vi "GUI.vi"(8 "error in (no error)":errorcluster) -> (0 "error out":errorcluster)   [LabVIEW 2017]
uses:
  Type Definitions/Queue FG Options.ctl
  Type Definitions/GUI Data.ctl
  Type Definitions/Controller States.ctl
  Type Definitions/Controller Message.ctl
  Type Definitions/Controller Data.ctl
  Type Definitions/DB Data.ctl
  Type Definitions/DB Info.ctl
  Type Definitions/Display Data.ctl
  Type Definitions/DB Record.ctl
  Type Definitions/Display Console States.ctl
  Type Definitions/Sensor UI Data.ctl
  Current State.vi
panel:
  in  "stop":bool
  in  "Transactions":T1
  in  "Pinpad":T2
  in  "Card Reader":bool
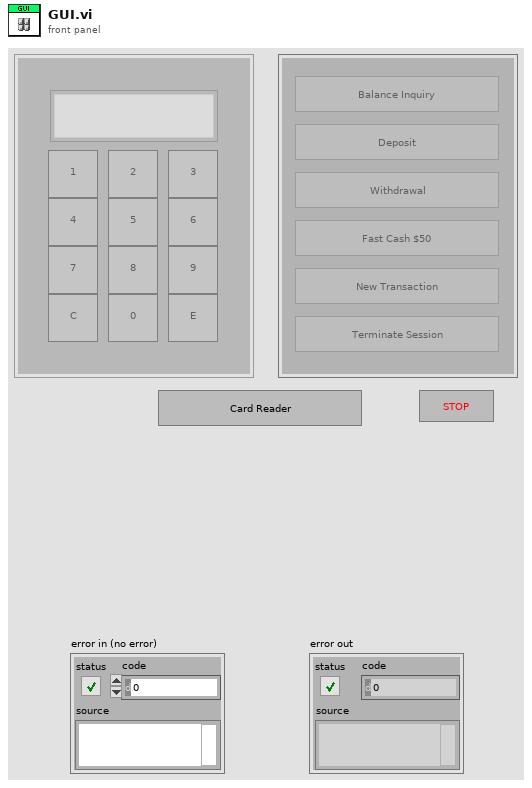
[diagram p1: front panel]
types:
  T1 = cluster{"Balance Inquiry":bool, "Deposit":bool, "Withdrawal":bool, "Fast Cash $50":bool, "New Transaction":bool, "Terminate Session":bool}
  T2 = cluster{"Screen":string, "num1":bool, "num2":bool, "num3":bool, "num6":bool, "num5":bool, "num4":bool, "num7":bool, "num8":bool, "num9":bool, "C":bool, "num0":bool, "E":bool}
  T3 = typedef "Queue FG Options.ctl" = enum16{"Set", "Get", "Read", "Write", "Destroy"}
  T4 = typedef "GUI Data.ctl" = cluster{"Card Reader":enum8{"Enabled", "Disabled", "Disabled and Grayed Out"}, "Keypad":enum8{"Enabled", "Disabled", "Disabled and Grayed Out"}, "Balance Inquiry":enum8{"Enabled", "Disabled", "Disabled and Grayed Out"}, "Deposit":enum8{"Enabled", "Disabled", "Disabled and Grayed Out"}, "Withdrawal":enum8{"Enabled", "Disabled", "Disabled and Grayed Out"}, "Fast Cash":enum8{"Enabled", "Disabled", "Disabled and Grayed Out"}, "New Transaction":enum8{"Enabled", "Disabled", "Disabled and Grayed Out"}, "Terminate Session":enum8{"Enabled", "Disabled", "Disabled and Grayed Out"}, "Pinpad Value":string, "Timeout":i32, "Controller States":T5}
  T5 = typedef "Controller States.ctl" = enum16{"Timeout", "Initial", "Login", "Idle", "Balance Inquiry", "Deposit", "Withdrawal", "Fast Cash", "Terminate", "Wait on Exit", "Shutdown", "Error Handler"}
  T6 = typedef "DB Info.ctl" = enum16{"Empty", "Verify", "Login Accepted", "Invalid Login", "Deposit Complete", "Withdrawal Complete", "Withdrawal Failed", "Terminate"}
  T7 = typedef "Controller Data.ctl" = cluster{"Time":dbl, "DB Data in":T8, "Display Data":T9, "GUI Data ":T4, "Sensor UI":T12, "Controller States":T5}
  T8 = typedef "DB Data.ctl" = cluster{"Account":i32, "First Name":string, "Last Name":string, "Balance":fxp<+/-,64,35>, "DB Info":T6}
  T9 = typedef "Display Data.ctl" = cluster{"Message Text":string, "DB Record":T10, "Card Read":bool, "Display Console States":T11}
  T10 = typedef "DB Record.ctl" = cluster{"Account":i32, "First Name":string, "Last Name":string, "Balance":fxp<+/-,64,35>}
  T11 = typedef "Display Console States.ctl" = enum16{"Timeout", "Initial", "Login", "Invalid Login", "Idle", "Balance Inquiry", "Deposit", "Withdrawal", "Fast Cash", "Withdrawal Failed", "Withdrawal Complete", "Terminate", "Shutdown"}
  T12 = typedef "Sensor UI Data.ctl" = cluster{"Funds dispensed":enum16{"Enabled", "Disabled", "Disabled and Grayed Out"}, "Deposit received":enum16{"Enabled", "Disabled", "Disabled and Grayed Out"}, "Timeout":dbl}
  T13 = typedef "Controller Message.ctl" = cluster{"Message Info":T5, "Message Data":variant}
  T14 = enum8{"Enabled", "Disabled", "Disabled and Grayed Out"}
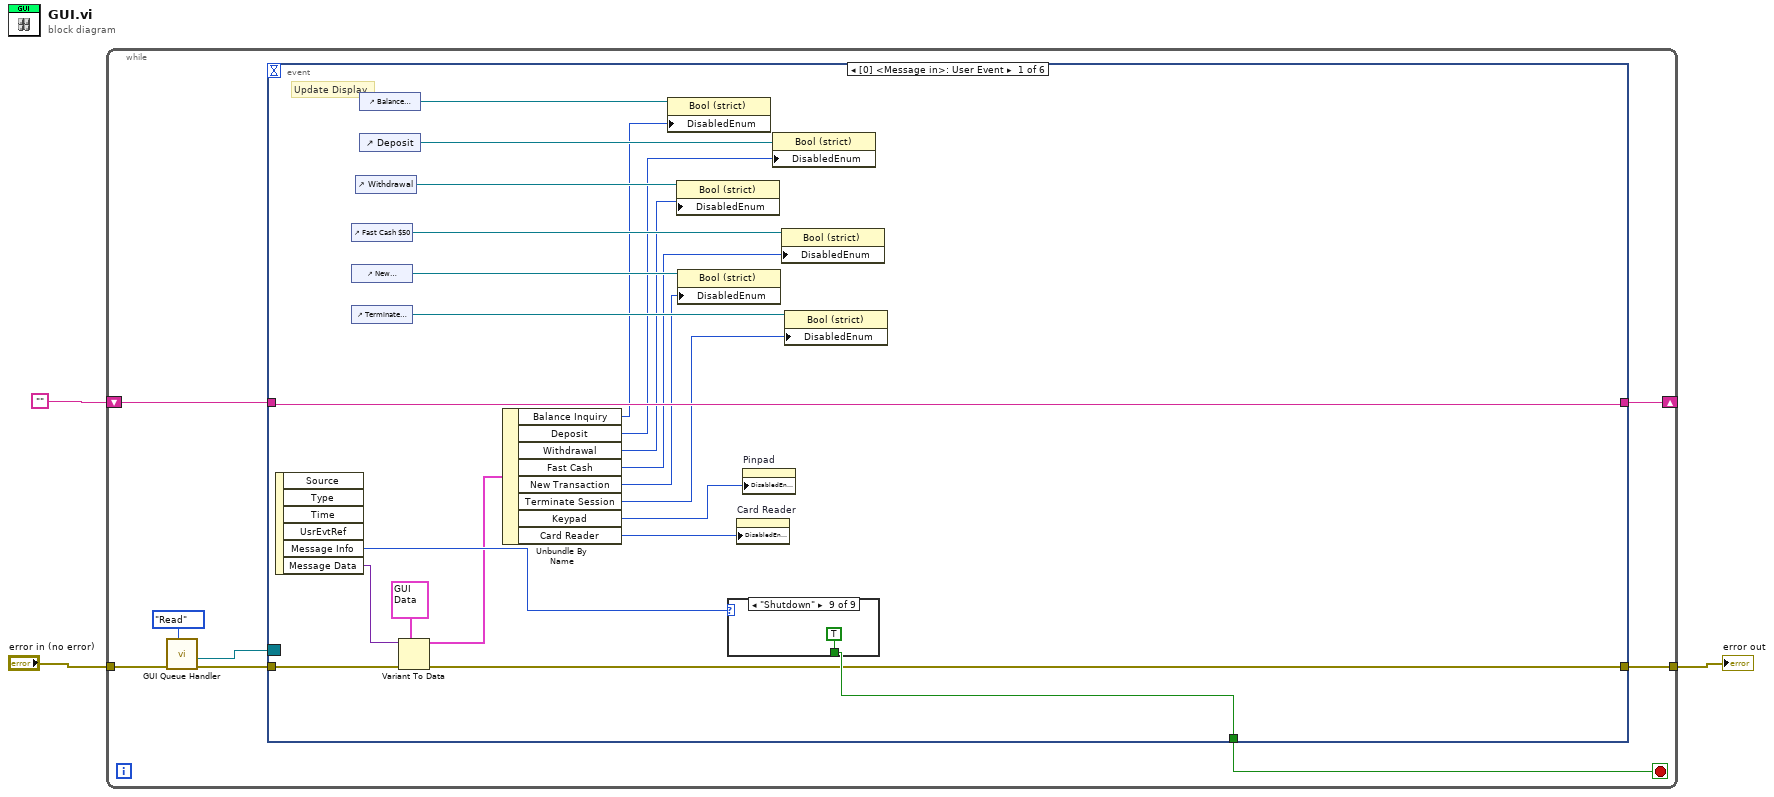
[diagram p0: block diagram]
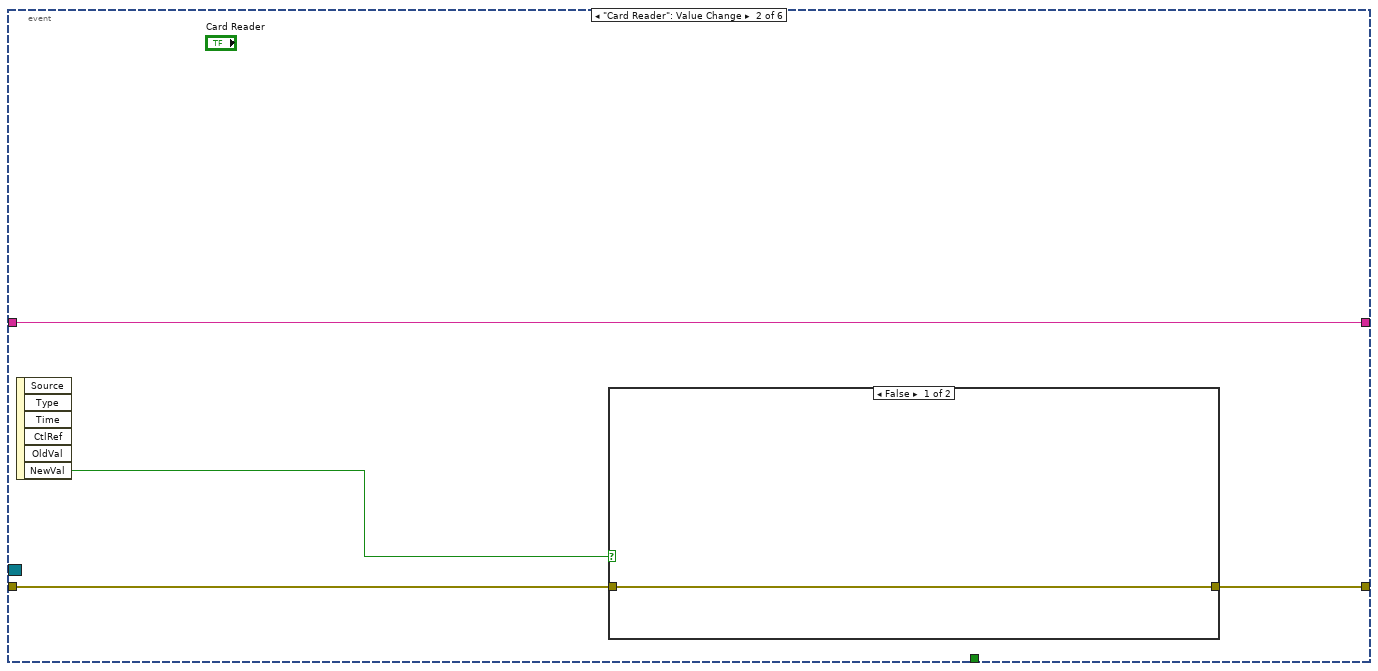
[diagram p10: hidden frame]
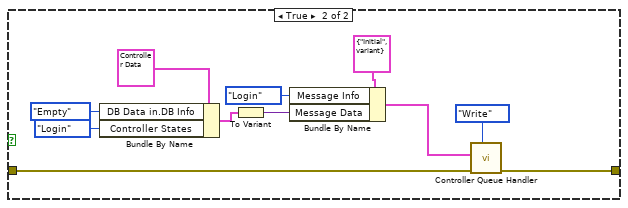
[diagram p11: hidden frame]
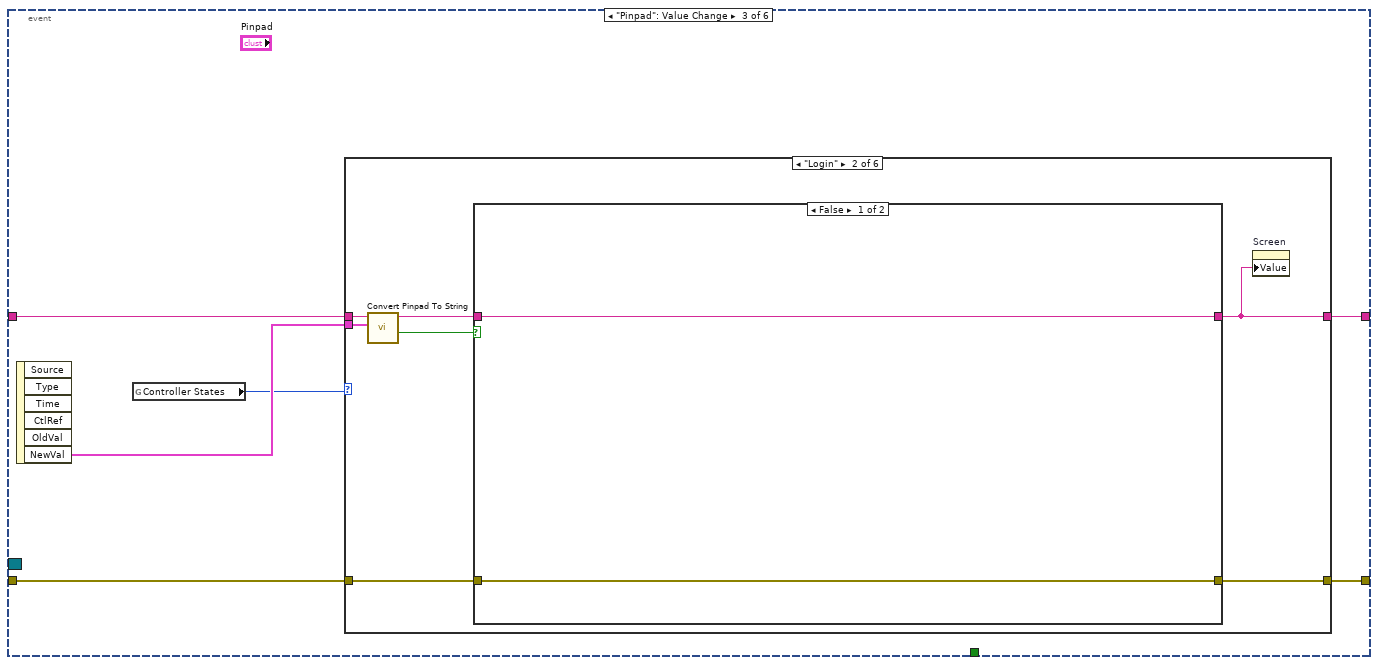
[diagram p12: hidden frame]
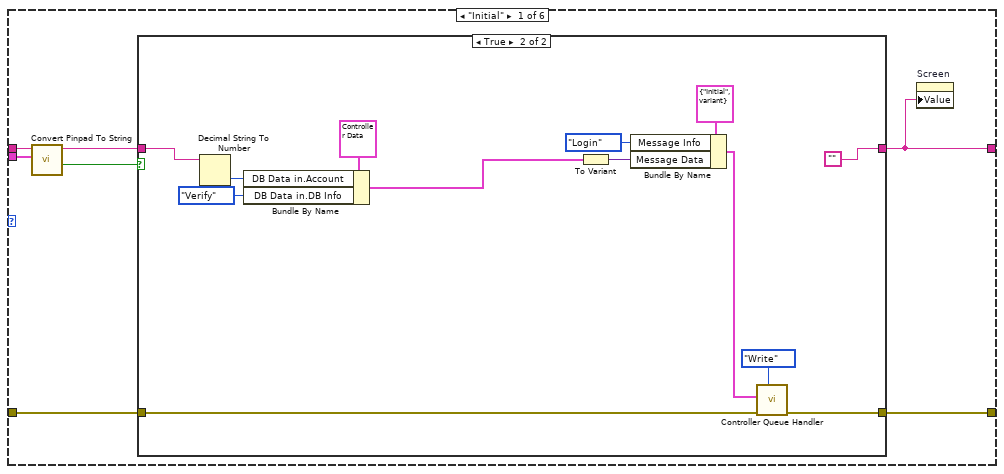
[diagram p13: hidden frame]
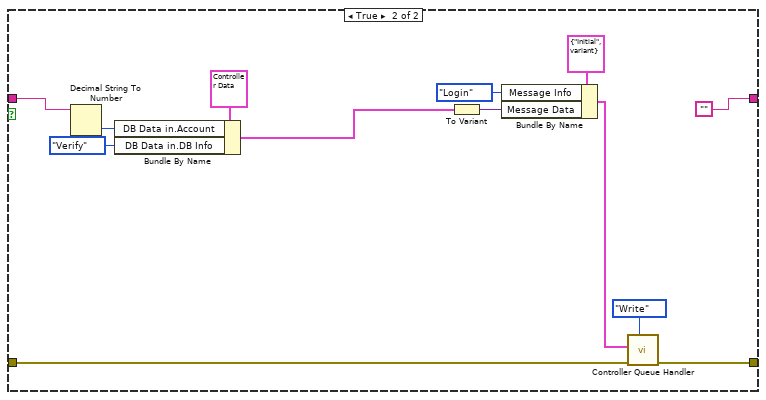
[diagram p15: hidden frame]
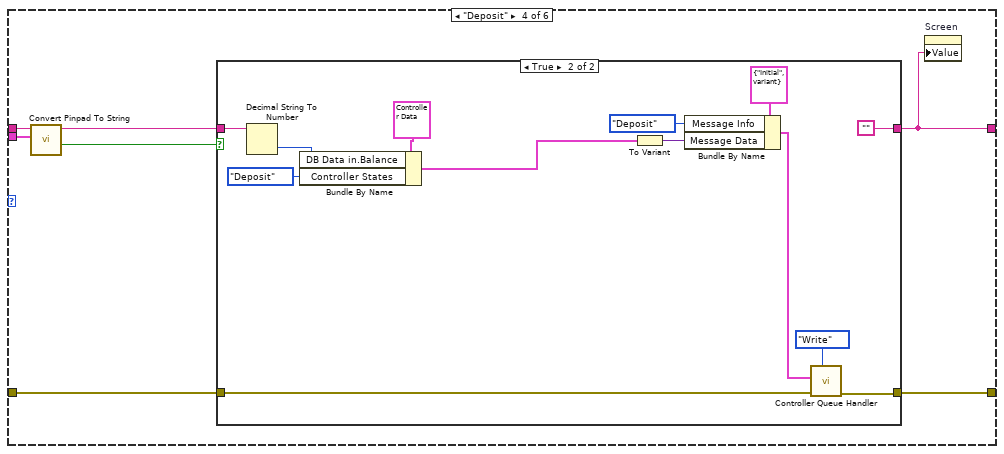
[diagram p17: hidden frame]
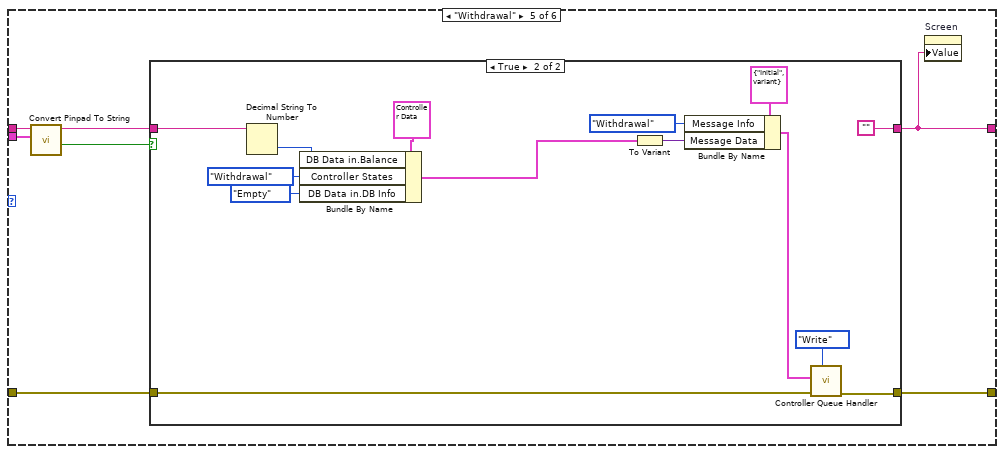
[diagram p19: hidden frame]
diagram:
  n1 = while {
    tunnel: "error in (no error)" -> [w6]
    tunnel: [w9] -> w2
    shift-right: [w7] -> _
    shift-left: "" -> [w8]
    stop <- w4 stop-if-true
    n2 = call "GUI Queue Handler.vi"("Action"=Queue_FG_Options."Read", "error in (no error)"=w6) -> ("error out"=w10:errorcluster, "Event Registration Refnum"=w5:refnum<event-registration>)  [unwired: 6 in, 2 out]
    n3 = event shown="[0] <Message in>: User Event" {
      selector: w5 -> [_ _ _ _ _ _]
      dyn-events: _ -> [_ _ _ _ _ _]
      timeout: _ -> [_ _ _ _ _ _]
      tunnel: w10 -> [w32 w37 w56 w157 w171 w240]
      tunnel: [w29 w36 w55 w154 w170 w240] -> w9
      tunnel: w8 -> [w33 w38 w54 w156 w169 w239]
      tunnel: [w33 w38 w53 w156 w168 w239] -> w7
      tunnel: [w30 _ _ TRUE _ _] -> w4
      event User Event {
        # "Update Display"
        n4 = event-data() -> ("Message Info"=w31:T5, "Message Data"=w28:variant)  [unwired: 1 in, 4 out]
        n5 = control-ref of="Fast Cash $50"() -> (w22:refnum<vi>)
        n6 = control-ref of="New Transaction"() -> (w21:refnum<vi>)
        n7 = control-ref of="Terminate Session"() -> (w20:refnum<vi>)
        n8 = control-ref of="Withdrawal"() -> (w19:refnum<vi>)
        n9 = control-ref of="Balance Inquiry"() -> (w24:refnum<vi>)
        n10 = control-ref of="Deposit"() -> (w23:refnum<vi>)
        n11 = Variant To Data(error in=w32, type=T4 {"Card Reader"=enum."Enabled", "Keypad"=enum."Enabled", "Balance Inquiry"=enum."Enabled", "Deposit"=enum."Enabled", "Withdrawal"=enum."Enabled", "Fast Cash"=enum."Enabled", "New Transaction"=enum."Enabled", "Terminate Session"=enum."Enabled", "Pinpad Value"="", "Timeout"=0, "Controller States"=enum."Initial"} ("GUI Data"), Variant=w28) -> (data=w26:T4, error out=w29:errorcluster)
        n12 = Unbundle By Name(w26) -> ("Balance Inquiry"=w17:T14, "Deposit"=w16:T14, "Withdrawal"=w14:T14, "Fast Cash"=w15:T14, "New Transaction"=w13:T14, "Terminate Session"=w12:T14, "Keypad"=w18:T14, "Card Reader"=w25:T14)
        n13 = property class="Bool (strict)"(reference=w24, "DisabledEnum"=w17) -> ()  [unwired: 1 in, 2 out]
        n14 = property class="Bool (strict)"(reference=w19, "DisabledEnum"=w14) -> ()  [unwired: 1 in, 2 out]
        n15 = property class="Bool (strict)"(reference=w21, "DisabledEnum"=w13) -> ()  [unwired: 1 in, 2 out]
        n16 = case shown="\"Shutdown\"" w31 {
          tunnel: [_ _ _ _ _ _ _ _ TRUE] -> w30
          frame "Initial", Default {
          }
          frame "Login" {
          }
          frame "Idle" {
          }
          frame "Balance Inquiry" {
          }
          frame "Deposit" {
          }
          frame "Withdrawal" {
          }
          frame "Fast Cash" {
          }
          frame "Terminate" {
          }
          frame "Shutdown" {
          }
        }
        n17 = property on="Card Reader" class="Bool"("DisabledEnum"=w25) -> ()  [unwired: 2 in, 2 out]
        n18 = property on="Pinpad" class="Clust (strict)"("DisabledEnum"=w18) -> ()  [unwired: 2 in, 2 out]
        n19 = property class="Bool (strict)"(reference=w23, "DisabledEnum"=w16) -> ()  [unwired: 1 in, 2 out]
        n20 = property class="Bool (strict)"(reference=w22, "DisabledEnum"=w15) -> ()  [unwired: 1 in, 2 out]
        n21 = property class="Bool (strict)"(reference=w20, "DisabledEnum"=w12) -> ()  [unwired: 1 in, 2 out]
      }
      event "Card Reader": Value Change {
        n22 = event-data() -> ("NewVal"=w35:bool)  [unwired: 1 in, 5 out]
        n23 = case shown="False" w35 {
          tunnel: w37 -> [w39 w50]
          tunnel: [w39 w49] -> w36
          frame False {
          }
          frame True {
            n24 = Bundle By Name(cluster=T7 {"Time"=0.0, "DB Data in"={"Account"=0, "First Name"="", "Last Name"="", "Balance"=0.0, "DB Info"=enum."Login Accepted"}, "Display Data"={"Message Text"="", "DB Record"={"Account"=0, "First Name"="", "Last Name"="", "Balance"=0.0}, "Card Read"=FALSE, "Display Console States"=enum."Timeout"}, "GUI Data "={"Card Reader"=enum."Enabled", "Keypad"=enum."Enabled", "Balance Inquiry"=enum."Enabled", "Deposit"=enum."Enabled", "Withdrawal"=enum."Enabled", "Fast Cash"=enum."Enabled", "New Transaction"=enum."Enabled", "Terminate Session"=enum."Enabled", "Pinpad Value"="", "Timeout"=0, "Controller States"=enum."Initial"}, "Sensor UI"={"Funds dispensed"=enum."Enabled", "Deposit received"=enum."Enabled", "Timeout"=0.0}, "Controller States"=enum."Timeout"} ("Controller Data"), "DB Data in.DB Info"=DB_Info."Empty", "Controller States"=Controller_States."Login") -> (w43:T7)
            n25 = To Variant(anything=w43) -> (Variant=w42:variant)
            n26 = Bundle By Name(cluster=T13 {"Message Info"=enum."Initial", "Message Data"=variant} ("Message"), "Message Info"=Controller_States."Login", "Message Data"=w42) -> (w45:T13)
            n27 = call "Controller Queue Handler.vi"("Action"=Queue_FG_Options."Write", "error in (no error)"=w50, "Message in"=w45) -> ("error out"=w49:errorcluster)  [unwired: 6 in, 2 out]
          }
        }
      }
      event "Pinpad": Value Change {
        n28 = event-data() -> ("NewVal"=w52:T2)  [unwired: 1 in, 5 out]
        n29 = global read "Current State.vi" "Controller States"() -> (w51:T5)
        n30 = case shown="\"Login\"" w51 {
          tunnel: w56 -> [w63 w85 w102 w106 w128 w149]
          tunnel: [w62 w84 w102 w105 w127 w149] -> w55
          tunnel: w54 -> [w61 w83 w101 w108 w130 w148]
          tunnel: [w59 w81 w101 w103 w125 w148] -> w53
          tunnel: w52 -> [w57 w79 _ w109 w131 _]
          frame "Initial" {
            n31 = call "Convert Pinpad To String.vi"("Pinpad"=w57, "Screen in"=w61) -> ("E"=w58:bool, "Screen out"=w60:string)  [unwired: 8 in]
            n32 = case shown="True" w58 {
              tunnel: w63 -> [w65 w76]
              tunnel: [w65 w73] -> w62
              tunnel: w60 -> [w64 w69]
              tunnel: [w64 ""] -> w59
              frame False {
              }
              frame True {
                n33 = Decimal String To Number(string=w69) -> (number=w68:i32)  [unwired: 2 in, 1 out]
                n34 = Bundle By Name(cluster=T7 {"Time"=0.0, "DB Data in"={"Account"=0, "First Name"="", "Last Name"="", "Balance"=0.0, "DB Info"=enum."Login Accepted"}, "Display Data"={"Message Text"="", "DB Record"={"Account"=0, "First Name"="", "Last Name"="", "Balance"=0.0}, "Card Read"=FALSE, "Display Console States"=enum."Timeout"}, "GUI Data "={"Card Reader"=enum."Enabled", "Keypad"=enum."Enabled", "Balance Inquiry"=enum."Enabled", "Deposit"=enum."Enabled", "Withdrawal"=enum."Enabled", "Fast Cash"=enum."Enabled", "New Transaction"=enum."Enabled", "Terminate Session"=enum."Enabled", "Pinpad Value"="", "Timeout"=0, "Controller States"=enum."Initial"}, "Sensor UI"={"Funds dispensed"=enum."Enabled", "Deposit received"=enum."Enabled", "Timeout"=0.0}, "Controller States"=enum."Timeout"} ("Controller Data"), "DB Data in.Account"=w68, "DB Data in.DB Info"=DB_Info."Verify") -> (w67:T7)
                n35 = To Variant(anything=w67) -> (Variant=w77:variant)
                n36 = Bundle By Name(cluster=T13 {"Message Info"=enum."Initial", "Message Data"=variant} ("Message"), "Message Info"=Controller_States."Login", "Message Data"=w77) -> (w71:T13)
                n37 = call "Controller Queue Handler.vi"("Action"=Queue_FG_Options."Write", "error in (no error)"=w76, "Message in"=w71) -> ("error out"=w73:errorcluster)  [unwired: 6 in, 2 out]
              }
            }
            n38 = property on="Screen" class="Str"("Value"=w59) -> ()  [unwired: 2 in, 2 out]
          }
          frame "Login" {
            n39 = call "Convert Pinpad To String.vi"("Pinpad"=w79, "Screen in"=w83) -> ("E"=w80:bool, "Screen out"=w82:string)  [unwired: 8 in]
            n40 = case shown="False" w80 {
              tunnel: w85 -> [w87 w98]
              tunnel: [w87 w95] -> w84
              tunnel: w82 -> [w86 w91]
              tunnel: [w86 ""] -> w81
              frame False {
              }
              frame True {
                n41 = Decimal String To Number(string=w91) -> (number=w90:i32)  [unwired: 2 in, 1 out]
                n42 = Bundle By Name(cluster=T7 {"Time"=0.0, "DB Data in"={"Account"=0, "First Name"="", "Last Name"="", "Balance"=0.0, "DB Info"=enum."Login Accepted"}, "Display Data"={"Message Text"="", "DB Record"={"Account"=0, "First Name"="", "Last Name"="", "Balance"=0.0}, "Card Read"=FALSE, "Display Console States"=enum."Timeout"}, "GUI Data "={"Card Reader"=enum."Enabled", "Keypad"=enum."Enabled", "Balance Inquiry"=enum."Enabled", "Deposit"=enum."Enabled", "Withdrawal"=enum."Enabled", "Fast Cash"=enum."Enabled", "New Transaction"=enum."Enabled", "Terminate Session"=enum."Enabled", "Pinpad Value"="", "Timeout"=0, "Controller States"=enum."Initial"}, "Sensor UI"={"Funds dispensed"=enum."Enabled", "Deposit received"=enum."Enabled", "Timeout"=0.0}, "Controller States"=enum."Timeout"} ("Controller Data"), "DB Data in.Account"=w90, "DB Data in.DB Info"=DB_Info."Verify") -> (w89:T7)
                n43 = To Variant(anything=w89) -> (Variant=w99:variant)
                n44 = Bundle By Name(cluster=T13 {"Message Info"=enum."Initial", "Message Data"=variant} ("Message"), "Message Info"=Controller_States."Login", "Message Data"=w99) -> (w93:T13)
                n45 = call "Controller Queue Handler.vi"("Action"=Queue_FG_Options."Write", "error in (no error)"=w98, "Message in"=w93) -> ("error out"=w95:errorcluster)  [unwired: 6 in, 2 out]
              }
            }
            n46 = property on="Screen" class="Str"("Value"=w81) -> ()  [unwired: 2 in, 2 out]
          }
          frame "Idle", Default {
          }
          frame "Deposit" {
            n47 = call "Convert Pinpad To String.vi"("Pinpad"=w109, "Screen in"=w108) -> ("E"=w107:bool, "Screen out"=w104:string)  [unwired: 8 in]
            n48 = case shown="True" w107 {
              tunnel: w106 -> [w110 w115]
              tunnel: [w110 w114] -> w105
              tunnel: w104 -> [w111 w116]
              tunnel: [w111 ""] -> w103
              frame False {
              }
              frame True {
                n49 = Decimal String To Number(string=w116) -> (number=w118:i32)  [unwired: 2 in, 1 out]
                n50 = Bundle By Name(cluster=T7 {"Time"=0.0, "DB Data in"={"Account"=0, "First Name"="", "Last Name"="", "Balance"=0.0, "DB Info"=enum."Login Accepted"}, "Display Data"={"Message Text"="", "DB Record"={"Account"=0, "First Name"="", "Last Name"="", "Balance"=0.0}, "Card Read"=FALSE, "Display Console States"=enum."Timeout"}, "GUI Data "={"Card Reader"=enum."Enabled", "Keypad"=enum."Enabled", "Balance Inquiry"=enum."Enabled", "Deposit"=enum."Enabled", "Withdrawal"=enum."Enabled", "Fast Cash"=enum."Enabled", "New Transaction"=enum."Enabled", "Terminate Session"=enum."Enabled", "Pinpad Value"="", "Timeout"=0, "Controller States"=enum."Initial"}, "Sensor UI"={"Funds dispensed"=enum."Enabled", "Deposit received"=enum."Enabled", "Timeout"=0.0}, "Controller States"=enum."Timeout"} ("Controller Data"), "DB Data in.Balance"=w118, "Controller States"=Controller_States."Deposit") -> (w117:T7)
                n51 = To Variant(anything=w117) -> (Variant=w123:variant)
                n52 = Bundle By Name(cluster=T13 {"Message Info"=enum."Initial", "Message Data"=variant} ("Message"), "Message Info"=Controller_States."Deposit", "Message Data"=w123) -> (w120:T13)
                n53 = call "Controller Queue Handler.vi"("Action"=Queue_FG_Options."Write", "error in (no error)"=w115, "Message in"=w120) -> ("error out"=w114:errorcluster)  [unwired: 6 in, 2 out]
              }
            }
            n54 = property on="Screen" class="Str"("Value"=w103) -> ()  [unwired: 2 in, 2 out]
          }
          frame "Withdrawal" {
            n55 = call "Convert Pinpad To String.vi"("Pinpad"=w131, "Screen in"=w130) -> ("E"=w129:bool, "Screen out"=w126:string)  [unwired: 8 in]
            n56 = case shown="True" w129 {
              tunnel: w128 -> [w132 w138]
              tunnel: [w132 w137] -> w127
              tunnel: w126 -> [w133 w139]
              tunnel: [w133 ""] -> w125
              frame False {
              }
              frame True {
                n57 = Decimal String To Number(string=w139) -> (number=w141:i32)  [unwired: 2 in, 1 out]
                n58 = Bundle By Name(cluster=T7 {"Time"=0.0, "DB Data in"={"Account"=0, "First Name"="", "Last Name"="", "Balance"=0.0, "DB Info"=enum."Login Accepted"}, "Display Data"={"Message Text"="", "DB Record"={"Account"=0, "First Name"="", "Last Name"="", "Balance"=0.0}, "Card Read"=FALSE, "Display Console States"=enum."Timeout"}, "GUI Data "={"Card Reader"=enum."Enabled", "Keypad"=enum."Enabled", "Balance Inquiry"=enum."Enabled", "Deposit"=enum."Enabled", "Withdrawal"=enum."Enabled", "Fast Cash"=enum."Enabled", "New Transaction"=enum."Enabled", "Terminate Session"=enum."Enabled", "Pinpad Value"="", "Timeout"=0, "Controller States"=enum."Initial"}, "Sensor UI"={"Funds dispensed"=enum."Enabled", "Deposit received"=enum."Enabled", "Timeout"=0.0}, "Controller States"=enum."Timeout"} ("Controller Data"), "DB Data in.Balance"=w141, "Controller States"=Controller_States."Withdrawal", "DB Data in.DB Info"=DB_Info."Empty") -> (w140:T7)
                n59 = To Variant(anything=w140) -> (Variant=w146:variant)
                n60 = Bundle By Name(cluster=T13 {"Message Info"=enum."Initial", "Message Data"=variant} ("Message"), "Message Info"=Controller_States."Withdrawal", "Message Data"=w146) -> (w143:T13)
                n61 = call "Controller Queue Handler.vi"("Action"=Queue_FG_Options."Write", "error in (no error)"=w138, "Message in"=w143) -> ("error out"=w137:errorcluster)  [unwired: 6 in, 2 out]
              }
            }
            n62 = property on="Screen" class="Str"("Value"=w125) -> ()  [unwired: 2 in, 2 out]
          }
          frame "Balance Inquiry" {
          }
        }
      }
      event "stop": Value Change {
        n63 = event-data() -> ()  [unwired: 1 in, 6 out]
        n64 = Bundle By Name(cluster=T13 {"Message Info"=enum."Initial", "Message Data"=variant} ("Message"), "Message Info"=Controller_States."Wait on Exit" ("Controller States")) -> (w151:T13)
        n65 = call "Controller Queue Handler.vi"("Action"=Queue_FG_Options."Write", "error in (no error)"=w157, "Message in"=w151) -> ("error out"=w154:errorcluster)  [unwired: 6 in, 2 out]
      }
      event "Transactions": Value Change {
        n66 = event-data() -> ("OldVal"=w158:T1, "NewVal"=w167:T1)  [unwired: 1 in, 4 out]
        n67 = Cluster To Array(cluster=w158) -> (array=w164:bool[])
        n68 = Cluster To Array(cluster=w167) -> (array=w166:bool[])
        n69 = Search 1D Array(1D array=w164, element=TRUE) -> (index of element=w161:i32)  [unwired: 1 in]
        n70 = Search 1D Array(1D array=w166, element=TRUE) -> (index of element=w159:i32)  [unwired: 1 in]
        n71 = Equal?(x=w159, y=-1) -> (x = y?=w162:bool)
        n72 = Select(t=w161, s=w162, f=w159) -> (s? t:f=w160:i32)
        n73 = case shown="1" w160 {
          tunnel: w171 -> [w183 w194 w205 w216 w227 w238]
          tunnel: [w181 w192 w203 w214 w225 w236] -> w170
          tunnel: w169 -> [w182 w193 w204 w215 w226 w237]
          tunnel: [w182 w193 w204 w215 w226 w237] -> w168
          frame 0, Default {
            n74 = Bundle By Name(cluster=T7 {"Time"=0.0, "DB Data in"={"Account"=0, "First Name"="", "Last Name"="", "Balance"=0.0, "DB Info"=enum."Login Accepted"}, "Display Data"={"Message Text"="", "DB Record"={"Account"=0, "First Name"="", "Last Name"="", "Balance"=0.0}, "Card Read"=FALSE, "Display Console States"=enum."Timeout"}, "GUI Data "={"Card Reader"=enum."Enabled", "Keypad"=enum."Enabled", "Balance Inquiry"=enum."Enabled", "Deposit"=enum."Enabled", "Withdrawal"=enum."Enabled", "Fast Cash"=enum."Enabled", "New Transaction"=enum."Enabled", "Terminate Session"=enum."Enabled", "Pinpad Value"="", "Timeout"=0, "Controller States"=enum."Initial"}, "Sensor UI"={"Funds dispensed"=enum."Enabled", "Deposit received"=enum."Enabled", "Timeout"=0.0}, "Controller States"=enum."Timeout"} ("Controller Data"), "Controller States"=Controller_States."Balance Inquiry") -> (w174:T7)
            n75 = To Variant(anything=w174) -> (Variant=w173:variant)
            n76 = Bundle By Name(cluster=T13 {"Message Info"=enum."Initial", "Message Data"=variant} ("Message"), "Message Info"=Controller_States."Balance Inquiry", "Message Data"=w173) -> (w178:T13)
            n77 = call "Controller Queue Handler.vi"("Action"=Queue_FG_Options."Write", "error in (no error)"=w183, "Message in"=w178) -> ("error out"=w181:errorcluster)  [unwired: 6 in, 2 out]
          }
          frame 1 {
            n78 = Bundle By Name(cluster=T7 {"Time"=0.0, "DB Data in"={"Account"=0, "First Name"="", "Last Name"="", "Balance"=0.0, "DB Info"=enum."Login Accepted"}, "Display Data"={"Message Text"="", "DB Record"={"Account"=0, "First Name"="", "Last Name"="", "Balance"=0.0}, "Card Read"=FALSE, "Display Console States"=enum."Timeout"}, "GUI Data "={"Card Reader"=enum."Enabled", "Keypad"=enum."Enabled", "Balance Inquiry"=enum."Enabled", "Deposit"=enum."Enabled", "Withdrawal"=enum."Enabled", "Fast Cash"=enum."Enabled", "New Transaction"=enum."Enabled", "Terminate Session"=enum."Enabled", "Pinpad Value"="", "Timeout"=0, "Controller States"=enum."Initial"}, "Sensor UI"={"Funds dispensed"=enum."Enabled", "Deposit received"=enum."Enabled", "Timeout"=0.0}, "Controller States"=enum."Timeout"} ("Controller Data"), "Controller States"=Controller_States."Deposit") -> (w185:T7)
            n79 = To Variant(anything=w185) -> (Variant=w184:variant)
            n80 = Bundle By Name(cluster=T13 {"Message Info"=enum."Initial", "Message Data"=variant} ("Message"), "Message Info"=Controller_States."Deposit", "Message Data"=w184) -> (w189:T13)
            n81 = call "Controller Queue Handler.vi"("Action"=Queue_FG_Options."Write", "error in (no error)"=w194, "Message in"=w189) -> ("error out"=w192:errorcluster)  [unwired: 6 in, 2 out]
          }
          frame 2 {
            n82 = Bundle By Name(cluster=T7 {"Time"=0.0, "DB Data in"={"Account"=0, "First Name"="", "Last Name"="", "Balance"=0.0, "DB Info"=enum."Login Accepted"}, "Display Data"={"Message Text"="", "DB Record"={"Account"=0, "First Name"="", "Last Name"="", "Balance"=0.0}, "Card Read"=FALSE, "Display Console States"=enum."Timeout"}, "GUI Data "={"Card Reader"=enum."Enabled", "Keypad"=enum."Enabled", "Balance Inquiry"=enum."Enabled", "Deposit"=enum."Enabled", "Withdrawal"=enum."Enabled", "Fast Cash"=enum."Enabled", "New Transaction"=enum."Enabled", "Terminate Session"=enum."Enabled", "Pinpad Value"="", "Timeout"=0, "Controller States"=enum."Initial"}, "Sensor UI"={"Funds dispensed"=enum."Enabled", "Deposit received"=enum."Enabled", "Timeout"=0.0}, "Controller States"=enum."Timeout"} ("Controller Data"), "Controller States"=Controller_States."Withdrawal") -> (w196:T7)
            n83 = To Variant(anything=w196) -> (Variant=w195:variant)
            n84 = Bundle By Name(cluster=T13 {"Message Info"=enum."Initial", "Message Data"=variant} ("Message"), "Message Info"=Controller_States."Withdrawal", "Message Data"=w195) -> (w200:T13)
            n85 = call "Controller Queue Handler.vi"("Action"=Queue_FG_Options."Write", "error in (no error)"=w205, "Message in"=w200) -> ("error out"=w203:errorcluster)  [unwired: 6 in, 2 out]
          }
          frame 3 {
            n86 = Bundle By Name(cluster=T7 {"Time"=0.0, "DB Data in"={"Account"=0, "First Name"="", "Last Name"="", "Balance"=0.0, "DB Info"=enum."Login Accepted"}, "Display Data"={"Message Text"="", "DB Record"={"Account"=0, "First Name"="", "Last Name"="", "Balance"=0.0}, "Card Read"=FALSE, "Display Console States"=enum."Timeout"}, "GUI Data "={"Card Reader"=enum."Enabled", "Keypad"=enum."Enabled", "Balance Inquiry"=enum."Enabled", "Deposit"=enum."Enabled", "Withdrawal"=enum."Enabled", "Fast Cash"=enum."Enabled", "New Transaction"=enum."Enabled", "Terminate Session"=enum."Enabled", "Pinpad Value"="", "Timeout"=0, "Controller States"=enum."Initial"}, "Sensor UI"={"Funds dispensed"=enum."Enabled", "Deposit received"=enum."Enabled", "Timeout"=0.0}, "Controller States"=enum."Timeout"} ("Controller Data"), "Controller States"=Controller_States."Fast Cash") -> (w207:T7)
            n87 = To Variant(anything=w207) -> (Variant=w206:variant)
            n88 = Bundle By Name(cluster=T13 {"Message Info"=enum."Initial", "Message Data"=variant} ("Message"), "Message Info"=Controller_States."Fast Cash", "Message Data"=w206) -> (w211:T13)
            n89 = call "Controller Queue Handler.vi"("Action"=Queue_FG_Options."Write", "error in (no error)"=w216, "Message in"=w211) -> ("error out"=w214:errorcluster)  [unwired: 6 in, 2 out]
          }
          frame 4 {
            n90 = Bundle By Name(cluster=T7 {"Time"=0.0, "DB Data in"={"Account"=0, "First Name"="", "Last Name"="", "Balance"=0.0, "DB Info"=enum."Login Accepted"}, "Display Data"={"Message Text"="", "DB Record"={"Account"=0, "First Name"="", "Last Name"="", "Balance"=0.0}, "Card Read"=FALSE, "Display Console States"=enum."Timeout"}, "GUI Data "={"Card Reader"=enum."Enabled", "Keypad"=enum."Enabled", "Balance Inquiry"=enum."Enabled", "Deposit"=enum."Enabled", "Withdrawal"=enum."Enabled", "Fast Cash"=enum."Enabled", "New Transaction"=enum."Enabled", "Terminate Session"=enum."Enabled", "Pinpad Value"="", "Timeout"=0, "Controller States"=enum."Initial"}, "Sensor UI"={"Funds dispensed"=enum."Enabled", "Deposit received"=enum."Enabled", "Timeout"=0.0}, "Controller States"=enum."Timeout"} ("Controller Data"), "Controller States"=Controller_States."Idle") -> (w218:T7)
            n91 = To Variant(anything=w218) -> (Variant=w217:variant)
            n92 = Bundle By Name(cluster=T13 {"Message Info"=enum."Initial", "Message Data"=variant} ("Message"), "Message Info"=Controller_States."Idle", "Message Data"=w217) -> (w222:T13)
            n93 = call "Controller Queue Handler.vi"("Action"=Queue_FG_Options."Write", "error in (no error)"=w227, "Message in"=w222) -> ("error out"=w225:errorcluster)  [unwired: 6 in, 2 out]
          }
          frame 5 {
            n94 = Bundle By Name(cluster=T7 {"Time"=0.0, "DB Data in"={"Account"=0, "First Name"="", "Last Name"="", "Balance"=0.0, "DB Info"=enum."Login Accepted"}, "Display Data"={"Message Text"="", "DB Record"={"Account"=0, "First Name"="", "Last Name"="", "Balance"=0.0}, "Card Read"=FALSE, "Display Console States"=enum."Timeout"}, "GUI Data "={"Card Reader"=enum."Enabled", "Keypad"=enum."Enabled", "Balance Inquiry"=enum."Enabled", "Deposit"=enum."Enabled", "Withdrawal"=enum."Enabled", "Fast Cash"=enum."Enabled", "New Transaction"=enum."Enabled", "Terminate Session"=enum."Enabled", "Pinpad Value"="", "Timeout"=0, "Controller States"=enum."Initial"}, "Sensor UI"={"Funds dispensed"=enum."Enabled", "Deposit received"=enum."Enabled", "Timeout"=0.0}, "Controller States"=enum."Timeout"} ("Controller Data"), "Controller States"=Controller_States."Terminate") -> (w229:T7)
            n95 = To Variant(anything=w229) -> (Variant=w228:variant)
            n96 = Bundle By Name(cluster=T13 {"Message Info"=enum."Initial", "Message Data"=variant} ("Message"), "Message Info"=Controller_States."Terminate", "Message Data"=w228) -> (w233:T13)
            n97 = call "Controller Queue Handler.vi"("Action"=Queue_FG_Options."Write", "error in (no error)"=w238, "Message in"=w233) -> ("error out"=w236:errorcluster)  [unwired: 6 in, 2 out]
          }
        }
      }
      event Timeout {
        n98 = event-data() -> ()  [unwired: 1 in, 3 out]
      }
    }
  }
  "error out" <- w2
